vi "ROI灰度分析.vi"() -> ()   [LabVIEW 2018]
uses:
  <vilib>/vision/NI_Vision_Development_Module.lvlib
panel:
  out "error out":errorcluster
  out "Image 2":T1(plugin-control)
  out "直方图":T2(graph)
  out "Image":T1(plugin-control)
  in  "路径":path
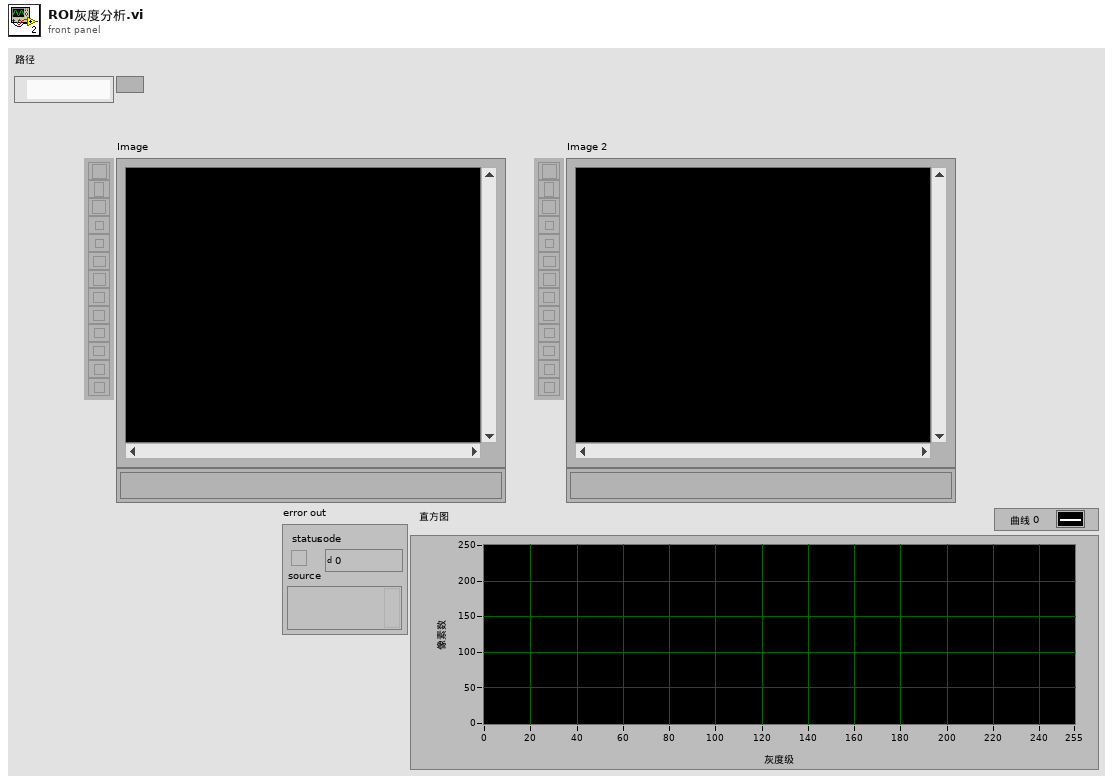
[diagram p1: front panel]
types:
  T1 = typedef "IMAQ Image.ctl" = refnum<image>
  T2 = cluster{"Starting Value":sgl, "Incremental Value":sgl, "Histogram":u32[]}
  T3 = typedef "Image Type" = u32
  T4 = typedef "IMAQ Rectangle" = cluster{"Left":i32, "Top":i32, "Right":i32, "Bottom":i32, "Rotation":dbl}
  T5 = typedef "ROI Descriptor" = cluster{"Global Rectangle":i32[], "Contours":cluster{"ID":enum32{"External", "Internal"}, "Type":u32, "Coordinates":i32[]}[]}
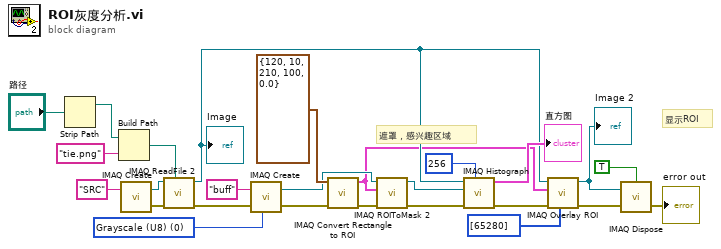
[diagram p0: block diagram]
diagram:
  w14 = T3 0 items=["Grayscale (U8)", "Grayscale (I16)", "Grayscale (SGL)", "Complex (CSG)", "RGB (U32)", "HSL (U32)", "RGB (U64)", "Grayscale (U16)"] ("Image Type")
  # "显示ROI"
  # "遮罩，感兴趣区域"
  n1 = Strip Path(path="路径") -> (stripped path=w25:path)  [unwired: 1 out]
  n2 = Build Path(base path=w25, name or relative path="tie.png" ("名称或相对路径")) -> (appended path=w19:path)
  n3 = call "IMAQ Create"("Image Name"="SRC") -> ("New Image"=w22:T1, "error out"=w21:errorcluster)  [unwired: 4 in]
  n4 = call "IMAQ ReadFile 2"("File Path"=w19, "error in (no error)"=w21, "Image"=w22) -> ("error out"=w12:errorcluster, "Image Out"=w9:T1)  [unwired: 4 in, 3 out]
  "Image" <- w9
  n5 = call "IMAQ Create"("Image Name"="buff", "Image Type"=w14, "error in (no error)"=w12) -> ("New Image"=w16:T1, "error out"=w18:errorcluster)  [unwired: 2 in]
  n6 = call "IMAQ Convert Rectangle to ROI"("error in (no error)"=w18, "Rectangle"=T4 {"Left"=120, "Top"=10, "Right"=210, "Bottom"=100, "Rotation"=0.0}) -> ("error out"=w15:errorcluster, "ROI Descriptor"=w8:T5)  [unwired: 7 in]
  n7 = call "IMAQ ROIToMask 2"("error in (no error)"=w15, "ROI Descriptor"=w8, "Image"=w16) -> ("error out"=w11:errorcluster, "Image Out"=w13:T1)  [unwired: 6 in, 1 out]
  n8 = call "IMAQ Histograph"("Number of Classes"=256, "error in (no error)"=w11, "Image Mask"=w13, "Image"=w9) -> ("error out"=w6:errorcluster, "Histogram Graph"=→"直方图":T2)  [unwired: 4 in, 2 out]
  n9 = call "IMAQ Overlay ROI"("Colors (Green)"=u32[] [65280], "error in (no error)"=w6, "ROI Descriptor"=w8, "Image"=w9) -> ("error out"=w4:errorcluster, "Image Out"=w3:T1)  [unwired: 6 in]
  "Image 2" <- w3
  n10 = call "IMAQ Dispose"("All Images? (No)"=TRUE, "Image"=w3, "error in (no error)"=w4) -> ("error out"=→"error out":errorcluster)  [unwired: 3 in]
